vi "Hue_Color_value.vi"(1 "Hue":dbl=350.7692307692308) -> (0 "Color":T1=enum."Blue")   [LabVIEW 2019]
uses:
  TypeDefs/ControlPanelColor.ctl
panel:
  in  "YellowTolerence":i32=40
  in  "YellowNominal":i32=60
  in  "RedTolerence":i32=10
  in  "RedNominal":i32=350
  in  "GreenTolerence":i32=10
  in  "GreenNominal":i32=180
  in  "BlueTolerence":i32=10
  in  "BlueNominal":i32=205
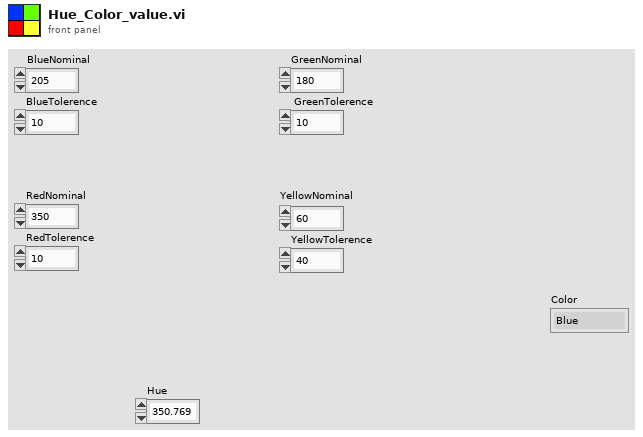
[diagram p1: front panel]
types:
  T1 = typedef "ControlPanelColor.ctl" = enum16{"Unknown", "Red", "Green", "Blue", "Yellow"}
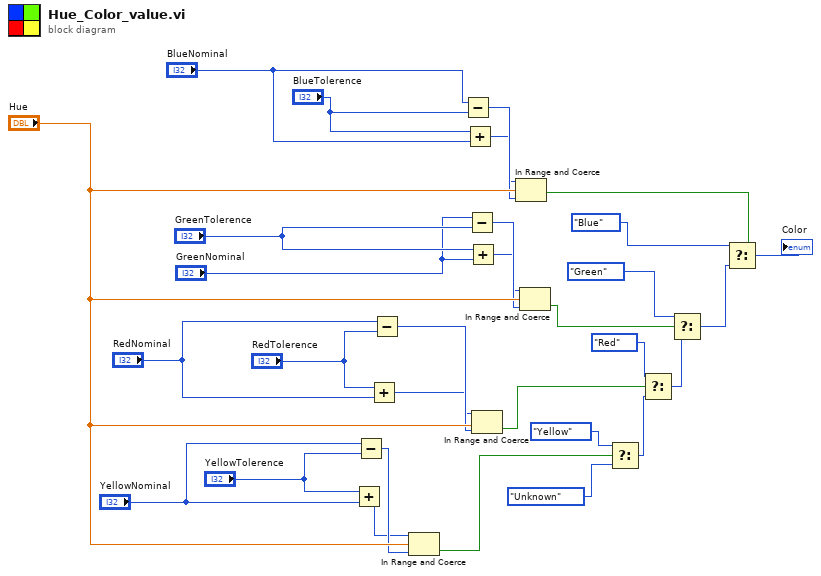
[diagram p0: block diagram]
diagram:
  n1 = Add(x="YellowTolerence", y="YellowNominal") -> (x+y=w1:i32)
  n2 = Subtract(x="YellowNominal", y="YellowTolerence") -> (x-y=w2:i32)
  n3 = Add(x="RedTolerence", y="RedNominal") -> (x+y=w3:i32)
  n4 = Subtract(x="RedNominal", y="RedTolerence") -> (x-y=w4:i32)
  n5 = In Range and Coerce(upper limit=w1, x="Hue", lower limit=w2) -> (In Range?=w19:bool)  [unwired: 1 out]
  n6 = Subtract(x="BlueNominal", y="BlueTolerence") -> (x-y=w13:i32)
  n7 = Add(x="BlueTolerence", y="BlueNominal") -> (x+y=w12:i32)
  n8 = Subtract(x="GreenNominal", y="GreenTolerence") -> (x-y=w6:i32)
  n9 = Add(x="GreenTolerence", y="GreenNominal") -> (x+y=w5:i32)
  n10 = In Range and Coerce(upper limit=w3, x="Hue", lower limit=w4) -> (In Range?=w21:bool)  [unwired: 1 out]
  n11 = In Range and Coerce(upper limit=w12, x="Hue", lower limit=w13) -> (In Range?=w23:bool)  [unwired: 1 out]
  n12 = In Range and Coerce(upper limit=w5, x="Hue", lower limit=w6) -> (In Range?=w22:bool)  [unwired: 1 out]
  n13 = Select(t=ControlPanelColor."Yellow", s=w19, f=ControlPanelColor."Unknown" ("Color 2")) -> (s? t:f=w30:T1)
  n14 = Select(t=ControlPanelColor."Red", s=w21, f=w30) -> (s? t:f=w29:T1)
  n15 = Select(t=ControlPanelColor."Green", s=w22, f=w29) -> (s? t:f=w28:T1)
  n16 = Select(t=ControlPanelColor."Blue", s=w23, f=w28) -> (s? t:f=→"Color":T1)
